vi "WPI_IMU_FGV.vi"(0 "ADI IMU Interrupt DevRef":T3={"ADI IMU DevRef"={"DevStatus"={"status"=FALSE, "code"=0, "source"=""}, "Handle"=0, "SPI Bus"=enum."SPI On-Board, CS0", "Device Found"=FALSE, "Device Ready"=FALSE, "Yaw Axis"=enum."Z", "AHRS Algorithm"=enum."Complementary"}, "InterruptRef"={"DevStatus"={"status"=FALSE, "code"=0, "source"=""}, "InterruptIndex"=enum."0"}}, 1 "Operation":enum16{"set", "get", "set reset"}(ring), 2 "Sensor Ready?":bool, 5 "Reset":bool, 7 "IMU Data":T8, 9 "IMU Angles":T1, 11 "IMU AHRS":cluster{"Pitch":dbl, "Roll":dbl, "Yaw":dbl}, 12 "IMU AHRS Delta":cluster{"Pitch":dbl, "Roll":dbl, "Yaw":dbl}) -> (4 "ADI IMU Interrupt DevRef Out":T3={"ADI IMU DevRef"={"DevStatus"={"status"=FALSE, "code"=0, "source"=""}, "Handle"=0, "SPI Bus"=enum."SPI On-Board, CS0", "Device Found"=FALSE, "Device Ready"=FALSE, "Yaw Axis"=enum."Z", "AHRS Algorithm"=enum."Complementary"}, "InterruptRef"={"DevStatus"={"status"=FALSE, "code"=0, "source"=""}, "InterruptIndex"=enum."0"}}, 6 "Reset Out":bool, 8 "IMU Data Out":T2, 10 "IMU Angles Out":T1, 13 "Sensor Ready Out":bool, 14 "IMU AHRS Delta Out":cluster{"Pitch":dbl, "Roll":dbl, "Yaw":dbl}, 15 "IMU AHRS Out":cluster{"Pitch":dbl, "Roll":dbl, "Yaw":dbl})   [LabVIEW 2015, in "FRC ADI MXP IMU.lvlib"]
uses:
  FRC ADI MXP IMU.lvlib
  WPI_AnalogDevicesIMUInterruptDevRef.ctl
  WPI_AnalogDevicesIMUDevRef.ctl
  <vilib>/Rock Robotics/SystemInterfaces/spilib/spi_bus.ctl
  <vilib>/Rock Robotics/WPI/Interrupt/WPI_InterruptRef.ctl
  <vilib>/Rock Robotics/SystemInterfaces/Interrupt/FPGA_InterruptIndex.ctl
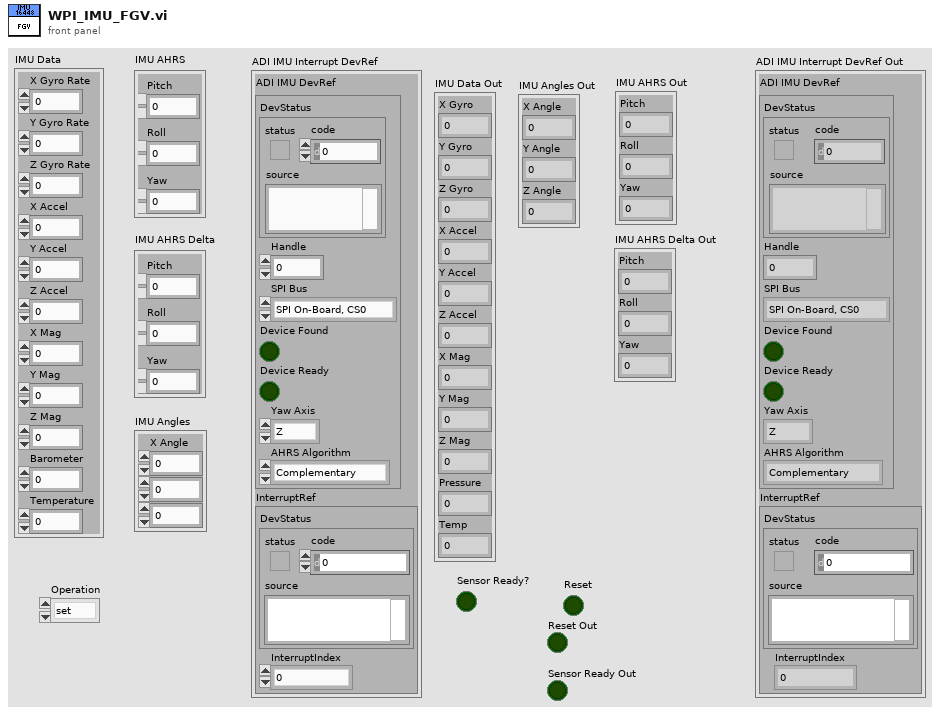
[diagram p1: front panel]
types:
  T1 = cluster{"X Angle":dbl, "Y Angle":dbl, "Z Angle":dbl}
  T2 = cluster{"X Gyro":dbl, "Y Gyro":dbl, "Z Gyro":dbl, "X Accel":dbl, "Y Accel":dbl, "Z Accel":dbl, "X Mag":dbl, "Y Mag":dbl, "Z Mag":dbl, "Pressure":dbl, "Temp":dbl}
  T3 = typedef "FRC ADI MXP IMU.lvlib/WPI_AnalogDevicesIMUInterruptDevRef.ctl" = cluster{"ADI IMU DevRef":T4, "InterruptRef":T6}
  T4 = typedef "FRC ADI MXP IMU.lvlib/WPI_AnalogDevicesIMUDevRef.ctl" = cluster{"DevStatus":errorcluster, "Handle":i32, "SPI Bus":T5, "Device Found":bool, "Device Ready":bool, "Yaw Axis":enum16{"X", "Y", "Z"}, "AHRS Algorithm":enum16{"Complementary", "Madgwick"}}
  T5 = typedef "spi_bus.ctl" = enum16{"SPI On-Board, CS0", "SPI On-Board, CS1", "SPI On-Board, CS2", "SPI On-Board, CS3", "SPI MXP", "Invalid"}
  T6 = typedef "WPI_InterruptRef.ctl" = cluster{"DevStatus":errorcluster, "InterruptIndex":T7}
  T7 = typedef "FPGA_InterruptIndex.ctl" = enum8{"0", "1", "2", "3", "4", "5", "6", "7", "Invalid"}
  T8 = cluster{"X Gyro Rate":dbl, "Y Gyro Rate":dbl, "Z Gyro Rate":dbl, "X Accel":dbl, "Y Accel":dbl, "Z Accel":dbl, "X Mag":dbl, "Y Mag":dbl, "Z Mag":dbl, "Barometer":dbl, "Temperature":dbl}
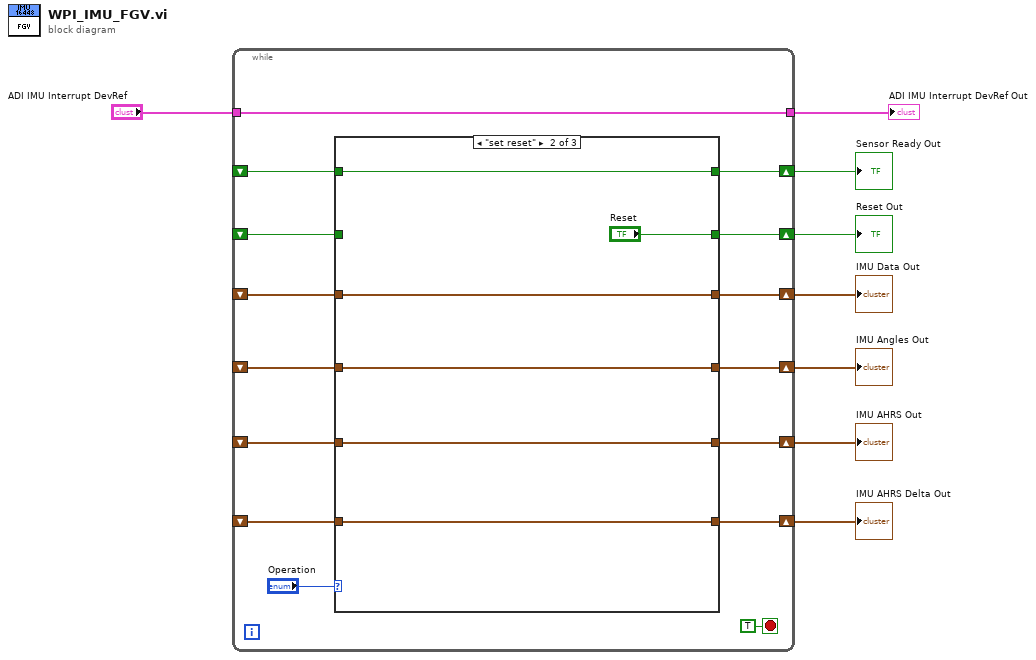
[diagram p0: block diagram]
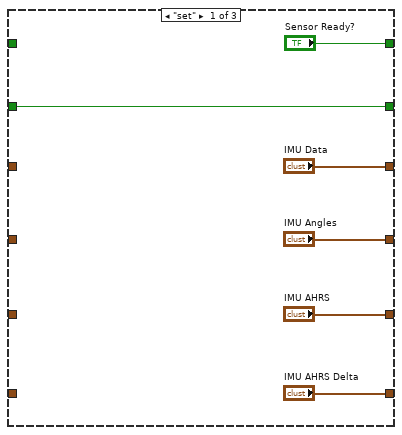
[diagram p2: hidden frame]
diagram:
  n1 = while {
    shift-right: [w21] -> w8
    shift-left: _ -> [w15]
    shift-right: [w20] -> w3
    shift-left: _ -> [w16]
    tunnel: "ADI IMU Interrupt DevRef" -> [w19]
    tunnel: [w19] -> w4
    shift-right: [w18] -> w2
    shift-left: _ -> [w17]
    shift-right: [w14] -> w1
    shift-left: _ -> [w13]
    shift-right: [w12] -> w7
    shift-left: _ -> [w11]
    shift-right: [w9] -> w6
    shift-left: _ -> [w10]
    stop <- TRUE stop-if-true
    n2 = case shown="\"set reset\"" "Operation" {
      tunnel: [w24 "Reset" w39] -> w21
      tunnel: ["IMU Data" w31 w40] -> w20
      tunnel: ["IMU Angles" w32 w41] -> w18
      tunnel: w17 -> [_ w32 w41]
      tunnel: w16 -> [_ w31 w40]
      tunnel: w15 -> [w24 _ w39]
      tunnel: ["IMU AHRS" w33 w38] -> w14
      tunnel: w13 -> [_ w33 w38]
      tunnel: ["IMU AHRS Delta" w34 w37] -> w12
      tunnel: w11 -> [_ w34 w37]
      tunnel: ["Sensor Ready?" w30 w36] -> w9
      tunnel: w10 -> [_ w30 w36]
      frame "set" {
      }
      frame "set reset" {
      }
      frame "get", Default {
      }
    }
  }
  "Reset Out" <- w8
  "IMU AHRS Delta Out" <- w7
  "Sensor Ready Out" <- w6
  "ADI IMU Interrupt DevRef Out" <- w4
  "IMU Data Out" <- w3
  "IMU Angles Out" <- w2
  "IMU AHRS Out" <- w1
